vi "Process.vi"(9 "process sync":refnum<notifier>, 11 "DAQ_Engine in":refnum<class "DAQ_Engine.lvclass">) -> ()   [LabVIEW 2019, in "DAQ_Engine.lvclass"]
doc: "Developed by Kevin Thompson\nkevin@thompsonengineering.net\n\nCopyright 2018\nThompson Engineering, LLC"
uses:
  DAQ_Engine.lvclass
  Common/DataTypes/Measurement Config--cluster.ctl
  DataTypes/DAQLoopSMcase--enum.ctl
  DataTypes/Process - AppData--cluster.ctl
  DataTypes/Settings--cluster.ctl
  Common/DataTypes/Acquisition Mode--cluster.ctl
  DataTypes/Dependency--cluster.ctl
  Config/Config.lvclass
  DataTypes/Public Events--cluster.ctl
  Common/DataTypes/TD Async CmdMsg EventData--cluster.ctl
  DataTypes/DAQStateChg EvData--cluster.ctl
  DataTypes/DAQStateEvData--cluster.ctl
  Common/DataTypes/DAQState--enum.ctl
  DataTypes/DAQMeasSettingsChg EvData--cluster.ctl
  DataTypes/DAQMeasSettingsEvData--cluster.ctl
  DataTypes/DAQAcqModeChg EvData--cluster.ctl
  Common/DataTypes/RawDAQDataQRef--cluster.ctl
  Common/DataTypes/RawDAQData--cluster.ctl
  Common/DataTypes/RawChannelData--cluster.ctl
  Common/DataTypes/TD GetSet ActionSelect--enum.ctl
  DAQ_Engine.lvclass/DAQ_Engine.ctl
  DataTypes/PrivateAsynEv_DAQ_Engine--enum.ctl
  Accessors/Get Settings.vi
  Accessors/Get PublicEvents.vi
  Accessors/Get Dependency.vi
  Accessors/Get RawDaqDataQRef.vi
  Accessors/Get ObjData.vi
  Accessors/Set MeasSettings.vi
  Accessors/Set InverterDataAcqMode.vi
  Accessors/Get MeasSettings.vi
  Accessors/Get InverterDataAcqMode.vi
  <vilib>/TELLC/SMQ/Add States to Queue using MultiLine String with vData.vi
  Common/Startup/GBL System.vi
panel:
  out "WaitFunction Value":u32
  out "computed loop time":u32
  out "ErrReporting":i32
  out "DAQ Error":bool
  out "DaqQ Timeout":bool
  in  "MeasSet":T1={"Data Rate 9775"=3.0, "Data Rate 9215"=1200000.0, "Samples RMS 9215"=480000, "Samples RMS 9775"=3}
  out "QuitSense":bool
  in  "HSLoopEn":bool
  in  "Enable DAQ":bool
  in  "Exit":bool
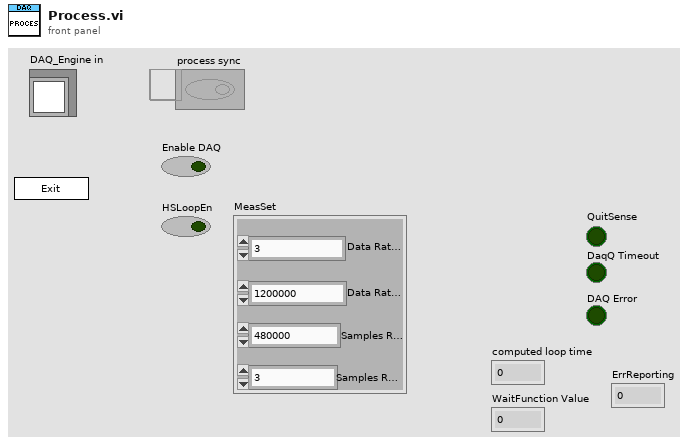
[diagram p1: front panel]
types:
  T1 = typedef "Measurement Config--cluster.ctl" = cluster{"Data Rate 9775":dbl, "Data Rate 9215":dbl, "Samples RMS 9215":u32, "Samples RMS 9775":u32}
  T2 = typedef "DAQ_Engine.lvclass/DAQLoopSMcase--enum.ctl" = enum16{"Init", "Run", "Stop"}
  T3 = typedef "TD GetSet ActionSelect--enum.ctl" = enum16{"Init", "Get", "Set"}
  T4 = typedef "DAQState--enum.ctl" = enum16{"Unknown", "Stopped", "Running", "Error"}
  T5 = typedef "DAQ_Engine.lvclass/Process - AppData--cluster.ctl" = cluster{"Core":cluster{"Current VI Reference":refnum<vi>, "Close Panel on Exit?":bool}, "Your Boolean data":bool, "Your string data":string, "SMQ":refnum<queue>, "Initialized?":bool, "Self Reference":refnum<class "DAQ_Engine.lvclass">, "Simulation?":bool, "process sync":refnum<notifier>, "vData":variant, "Settings":T6, "Dependency":T8, "Public Events":T9, "RawDaqDataQ":T10, "PrivateAsync Ev":refnum<user-event>, "MeasSet":T1, "AcqMode":T7, "DAQState Data":T11}
  T6 = typedef "DAQ_Engine.lvclass/Settings--cluster.ctl" = cluster{"Simulation":bool, "Initial ErrReporting setting":i32, "Initial Measurement settings":T1, "Acquisition mode":T7, "DemoMode":bool, "RIO Device":string}
  T7 = typedef "Acquisition Mode--cluster.ctl" = enum16{"3phase", "Single"}
  T8 = typedef "DAQ_Engine.lvclass/Dependency--cluster.ctl" = cluster{"Config":refnum<class "Config.lvclass">}
  T9 = typedef "DAQ_Engine.lvclass/Public Events--cluster.ctl" = cluster{"DAQ_Engine.AsyncCmd Event":refnum<user-event>, "DAQ_Engine.AsyncMsg Event":refnum<user-event>, "stop process":refnum<user-event>, "DAQ_Engine.DAQStateChg Ev":refnum<user-event>, "DAQ_Engine.MeasSettingsChg Ev":refnum<user-event>, "DAQ_Engine.AcqModeChg Ev":refnum<user-event>}
  T10 = typedef "RawDAQDataQRef--cluster.ctl" = refnum<queue>
  T11 = typedef "DAQ_Engine.lvclass/DAQStateEvData--cluster.ctl" = cluster{"DAQState":T4, "vData":variant}
  T12 = typedef "DAQ_Engine.lvclass/ObjData--cluster.ctl" = cluster{"Settings":T6, "Public Events":T9, "Dependency":T8, "ReadData-placeholder":T13, "VISA-placeholder":refnum<visa-resource-name>, "MeasSettings":T1, "InverterDataAcqMode":T7, "RawDaqDataQ":T10, "Private Events":T14, "DAQState Data":T11}
  T13 = typedef "DAQ_Engine.lvclass/Read Data--cluster.ctl" = cluster{"Data":dbl}
  T14 = typedef "DAQ_Engine.lvclass/Private Events--cluster.ctl" = cluster{"PrivateAsync Ev":refnum<user-event>}
  T15 = typedef "DAQ_Engine.lvclass/PrivateAsynEv_DAQ_Engine--enum.ctl" = enum16{"PrivDAQ.EnableDAQ", "PrivDAQ.ClearDAQError"}
  T16 = enum32{"invalid app kind", "Development System", "Run Time System", "Student Edition", "Embedded LabVIEW", "Evaluation", "Custom"}
  T17 = enum32{"Invalid", "Standard", "Closed", "Hidden", "Minimized", "Maximized"}
  T18 = typedef "DAQ_Engine.lvclass/AsynCmd_DAQ_Engine--enum.ctl" = enum16{"DAQ.EnableDAQ", "DAQ.ClearDAQError", "DAQ.SetMeasConfig", "DAQ.SetAcqMode", "DAQ.SetErrorReporting"}
  T19 = cluster{"Current VI Reference":refnum<vi>, "Close Panel on Exit?":bool}
  T20 = typedef "RawDAQData--cluster.ctl" = cluster{"Module1-2_9775":T21, "Module 3-4_9215":T21}
  T21 = typedef "RawChannelData--cluster.ctl" = cluster{"TS":timestamp, "ScanArray":dbl[]}
  T22 = typedef "nirio_resource_hc.ctl" = tag
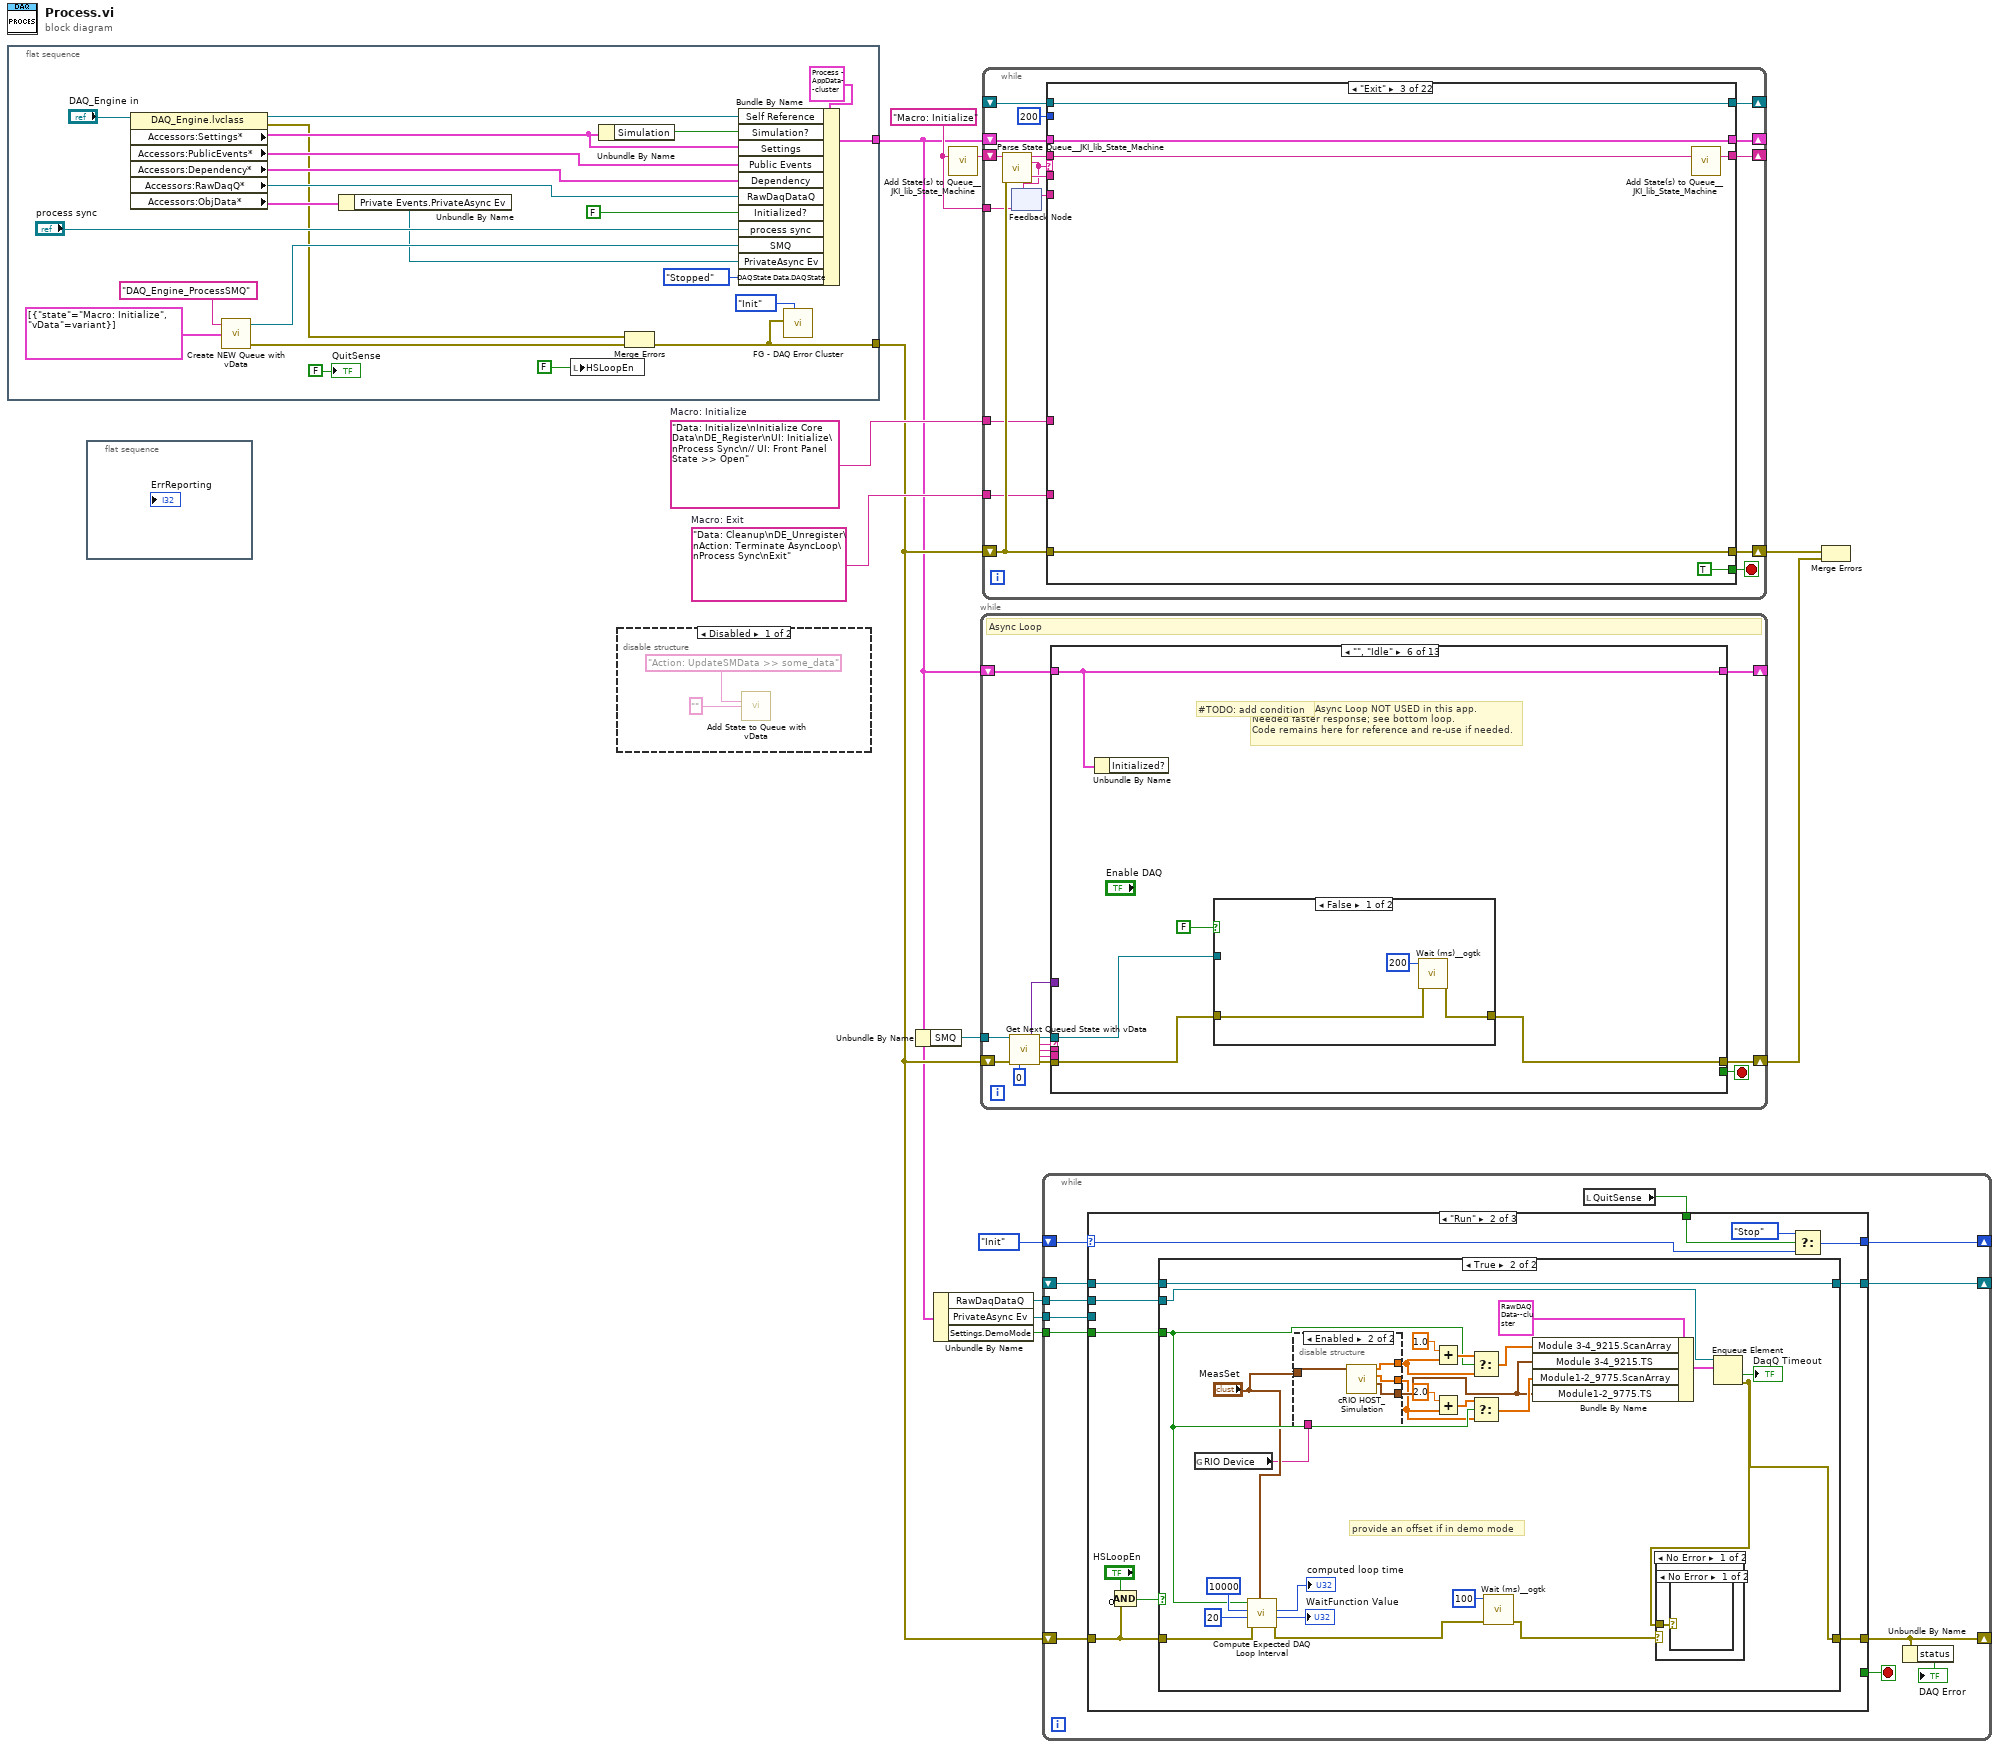
[diagram p0: block diagram]
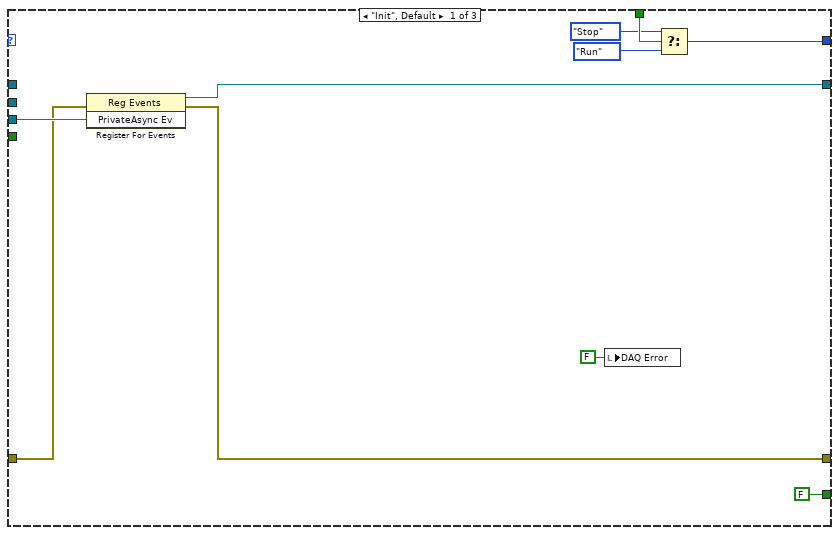
[diagram p2: hidden frame]
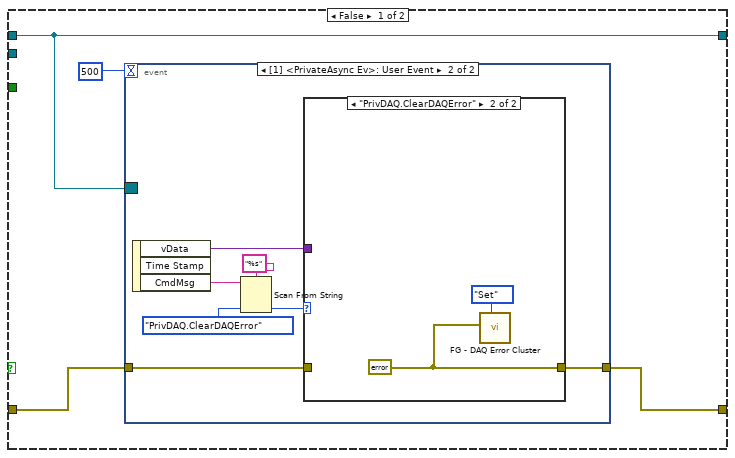
[diagram p3: hidden frame]
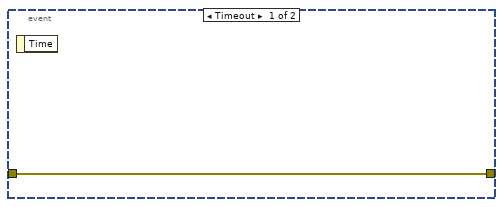
[diagram p4: hidden frame]
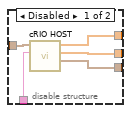
[diagram p6: hidden frame]
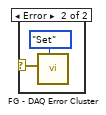
[diagram p7: hidden frame]
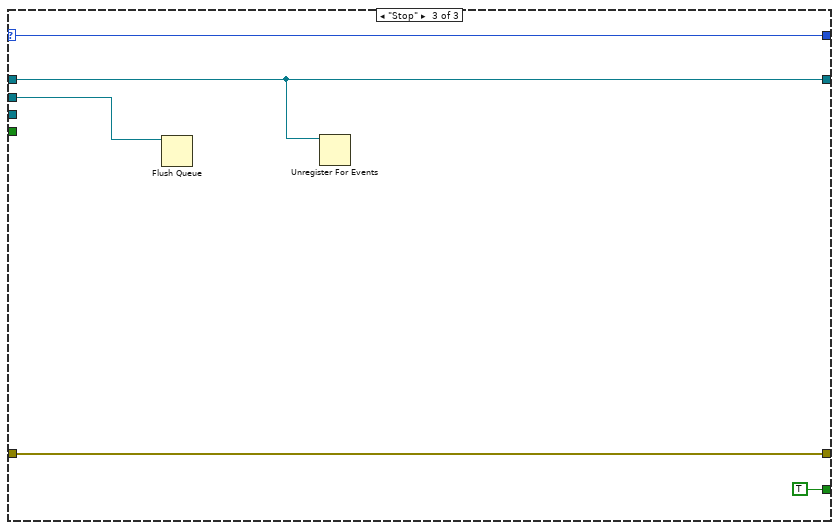
[diagram p9: hidden frame]
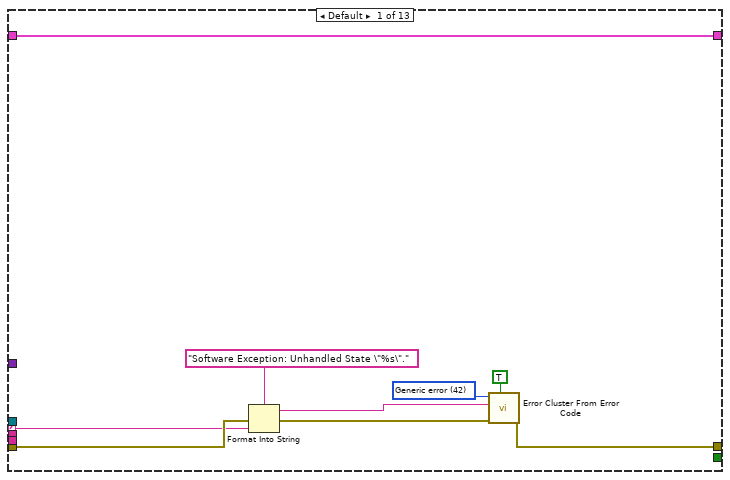
[diagram p11: hidden frame]
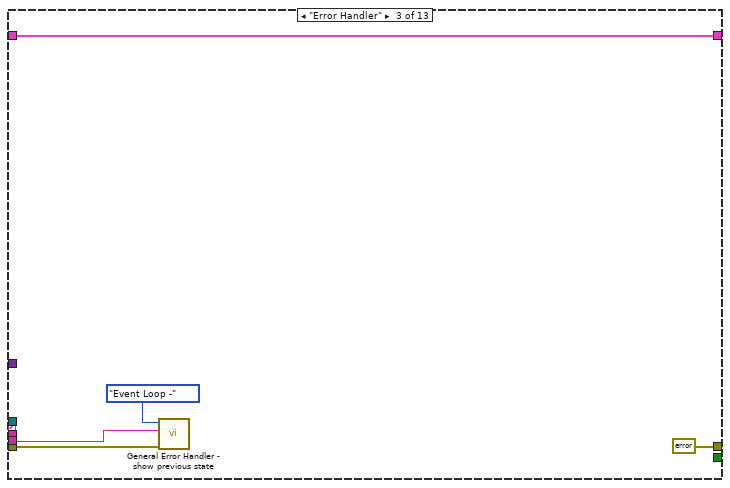
[diagram p13: hidden frame]
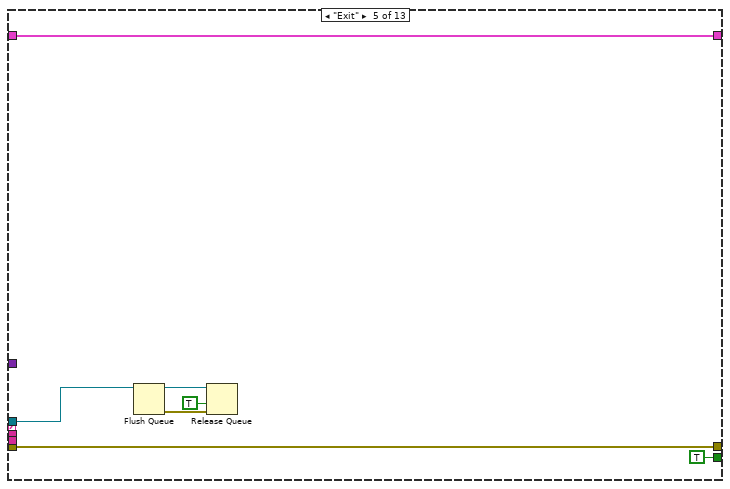
[diagram p15: hidden frame]
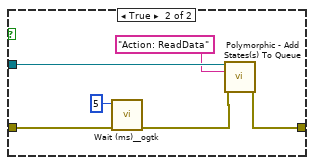
[diagram p16: hidden frame]
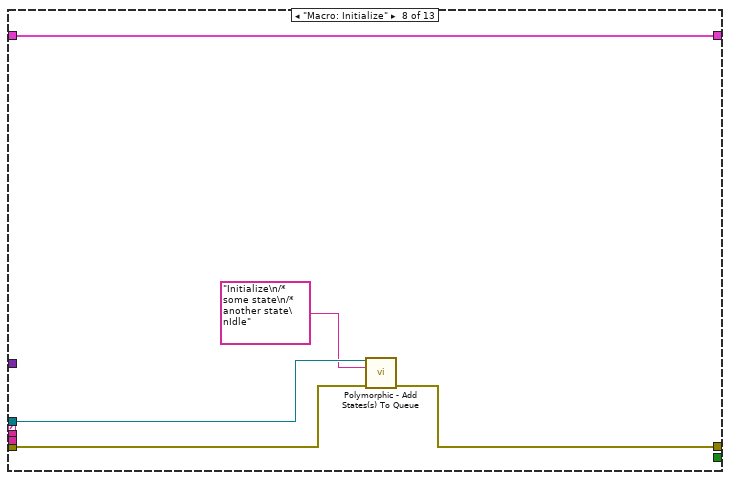
[diagram p18: hidden frame]
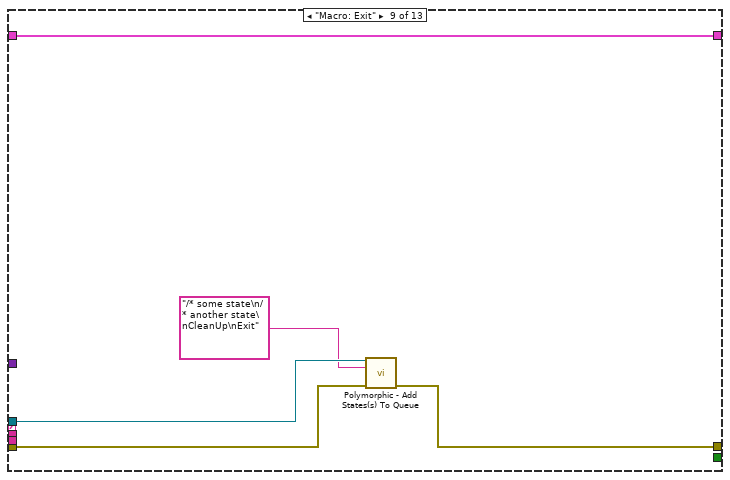
[diagram p19: hidden frame]
diagram:
  w11 = "Data: Cleanup\nDE_Unregister\nAction: Terminate AsyncLoop\nProcess Sync\nExit"  # Macro: Exit
  w12 = "Data: Initialize\nInitialize Core Data\nDE_Register\nUI: Initialize\nProcess Sync\n// UI: Front Panel State >> Open"  # Macro: Initialize
  w7 = "Macro: Initialize"
  n1 = flat-sequence {
    tunnel: [w36] -> w4
    tunnel: [w15] -> w5
    frame #0 {
      n2 = property class="DAQ_Engine.lvclass"(reference="DAQ_Engine in") -> (reference out=w17:refnum<class "DAQ_Engine.lvclass">, error out=w16:errorcluster, "Accessors:Settings*"=w27:T6, "Accessors:PublicEvents*"=w18:T9, "Accessors:Dependency*"=w29:T8, "Accessors:RawDaqQ*"=w23:T10, "Accessors:ObjData*"=w22:T12)  [unwired: 1 in]
      n3 = call <vilib>:"Create NEW Queue with vData.vi"("Initial States"=cluster{"state":string, "vData":variant}[] [{"state"="Macro: Initialize", "vData"=variant}], "Name (SMQ)"="DAQ_Engine_ProcessSMQ") -> ("error out"=w19:errorcluster, "queue out"=w35:refnum<queue>)  [unwired: 2 in]
      n4 = Unbundle By Name(w22) -> ("Private Events.PrivateAsync Ev"=w21:refnum<user-event>)
      n5 = local write "HSLoopEn"(FALSE ("HSLoopEn")) -> ()
      n6 = Unbundle By Name(w27) -> ("Simulation"=w28:bool)
      n7 = Merge Errors(w16, w19) -> (w15:errorcluster)
      n8 = Bundle By Name(cluster=T5 {"Core"={"Current VI Reference"=refnum, "Close Panel on Exit?"=FALSE}, "Your Boolean data"=FALSE, "Your string data"="", "SMQ"=refnum, "Initialized?"=FALSE, "Self Reference"=refnum, "Simulation?"=FALSE, "process sync"=refnum, "vData"=variant, "Settings"={"Simulation"=FALSE, "Initial ErrReporting setting"=0, "Initial Measurement settings"={"Data Rate 9775"=3.0, "Data Rate 9215"=1200000.0, "Samples RMS 9215"=480000, "Samples RMS 9775"=3}, "Acquisition mode"=enum."3phase", "DemoMode"=FALSE, "RIO Device"=""}, "Dependency"={"Config"=refnum}, "Public Events"={"DAQ_Engine.AsyncCmd Event"=refnum, "DAQ_Engine.AsyncMsg Event"=refnum, "stop process"=refnum, "DAQ_Engine.DAQStateChg Ev"=refnum, "DAQ_Engine.MeasSettingsChg Ev"=refnum, "DAQ_Engine.AcqModeChg Ev"=refnum}, "RawDaqDataQ"=refnum, "PrivateAsync Ev"=refnum, "MeasSet"={"Data Rate 9775"=3.0, "Data Rate 9215"=1200000.0, "Samples RMS 9215"=480000, "Samples RMS 9775"=3}, "AcqMode"=enum."3phase", "DAQState Data"={"DAQState"=enum."Unknown", "vData"=variant}} ("SM2 AppData"), "Self Reference"=w17, "Simulation?"=w28, "Settings"=w27, "Public Events"=w18, "Dependency"=w29, "RawDaqDataQ"=w23, "Initialized?"=FALSE, "process sync"="process sync", "SMQ"=w35, "PrivateAsync Ev"=w21, "DAQState Data.DAQState"=DAQState--enum."Stopped") -> (w36:T5)
      n9 = call "FG - DAQ Error Cluster.vi"("action (Get)"=TD_GetSet_ActionSelect--enum."Init", "error"=w15) -> ()  [unwired: 9 in, 1 out]
      "QuitSense" <- FALSE ("QuitSense")
    }
  }
  n10 = flat-sequence {
    frame #0 {
    }
  }
  n11 = disable-structure shown="Disabled" {
    frame Disabled {
      n12 = call <vilib>:"Add State to Queue with vData.vi"("state in"="Action: UpdateSMData >> some_data", "vData (\"\")"="") -> ()  [unwired: 10 in, 4 out]
    }
    frame Enabled {
    }
  }
  n13 = Unbundle By Name(w4) -> ("SMQ"=w10:refnum<queue>)
  n14 = Unbundle By Name(w4) -> ("RawDaqDataQ"=w6:T10, "PrivateAsync Ev"=w2:refnum<user-event>, "Settings.DemoMode"=w1:bool)
  n15 = call <vilib>:"Add State(s) to Queue__JKI_lib_State_Machine.vi"("State(s) in (\"\")"=w7) -> ("States Out"=w13:string)  [unwired: 14 in]
  n16 = while {
    shift-right: [w48] -> w8
    shift-left: w5 -> [w50]
    tunnel: w10 -> [w46]
    shift-right: [w44] -> _
    shift-left: w4 -> [w45]
    stop <- w39 stop-if-true
    # "Async Loop"
    n17 = call <vilib>:"Get Next Queued State with vData.vi"("queue in"=w46, "error in (no error)"=w50, "timeout (100)"=0) -> ("vData out"=w43:variant, "queue out"=w47:refnum<queue>, "Next State"=w51:string, "queued msg"=w41:string, "Prev State"=w40:string, "error out"=w49:errorcluster)  [unwired: 6 in, 1 out]
    n18 = case shown="\"\", \"Idle\"" w51 {
      tunnel: w47 -> [_ _ _ _ w70 w81 _ w96 w101 _ _ _ w120]
      tunnel: w41 -> [_ _ _ _ _ _ _ _ _ _ _ w109 w122]
      selector: w51 -> [w52 _ _ _ _ _ _ _ _ _ _ _ _]
      tunnel: w49 -> [w54 w62 w64 w69 w76 w78 w92 w95 w100 w104 w105 w108 w117]
      tunnel: [w53 w62 errorcluster {"status"=FALSE, "code"=0, "source"=""} ("error constant") w69 w76 w79 w92 w94 w99 w104 w105 w111 w116] -> w48
      tunnel: w45 -> [w60 w61 w67 w68 w75 w80 w91 w97 w102 w103 w106 w114 w119]
      tunnel: [w60 w61 w67 w68 w75 w80 w91 w97 w102 w103 w106 w114 w118] -> w44
      tunnel: w43 -> [_ _ _ _ _ _ _ _ _ _ _ _ w121]
      tunnel: w40 -> [_ _ w63 _ _ _ _ _ _ _ _ _ _]
      tunnel: [_ _ _ _ TRUE _ _ _ _ _ _ _ _] -> w39
      frame Default {
        w56 = 42 items=["No error", "Argument error", "Memory is full", "Out of zone", "End of file", "File already open", "Generic file I/O error", "File not found", "File permission error", "Disk is full", "Duplicate path", "Too many files open", "System feature not enabled", "Resource file not found", "Cannot add resource", "Resource not found", "Image not found", "Image memory error", "Pen does not exist", "Config type invalid", "Config token not found", "Config parse error", "Config memory error", "Bad external code format", "Bad external code offset", "External code not present", "Null window", "Destroy window error", "Null menu", "Print aborted", "Bad print record", "Print driver error", "Windows error during printing", "Memory error during printing", "Print dialog error", "Generic print error", "Invalid device refnum", "Device not found", "Device parameter error", "Device unit error", "Cannot open device", "Device call aborted", "Generic error", "Cancelled by user", "Object ID too low", "Object ID too high", "Object not in heap", "Unknown heap", "Unknown object (invalid DefProc)", "Unknown object (DefProc not in table)", "Message out of range", "Invalid (null) method", "Unknown message", "Manager call not supported", "Bad address", "Network operation in progress", "Network operation timed out", "Connection is busy", "Network attribute not supported", "Network error", "Address in use", "System out of memory", "Connection aborted", "Connection refused", "Not connected", "Already connected", "Connection closed", "Initialization error (interapplication manager)", "Bad occurrence", "Wait on unbound occurrence handler", "Occurrence queue overflow", "Datalog type conflict", "Unused", "Unrecognized type (interapplication manager)", "Memory corrupt", "Failed to make temporary DLL", "Old CIN version", "Drag socket not found", "Failed to load drop-object", "Failed to register OLE object", "Failed to release OLE object", "Format specifier type mismatch", "Unknown format specifier", "Too few format specifiers", "Too many format specifiers", "Scan failed", "Newer CIN version", "Error converting to variant", "Runtime menu error", "Password tampered", "Variant attribute not found", "Incompatible variant data type", "Event data is not available", "Event Store is not present", "Occurrence is not found", "Event Queue is not created", "Event info is not available", "Refnum passed is NULL", "Error retrieving Class GUID", "Error retrieving CoClass GUID", "Error retrieving TypeLib GUID.", "Bad built application magic bytes.", "Specific driver is different from the specific driver associated with the Logical Name.", "There is no session opened to the class driver.", "Max Error", "MAX - Error with config objects", "MAX - Error loading configuration", "MAX - Group not supported"]
        n19 = Format Into String(format string="Software Exception: Unhandled State \"%s\"." ("message"), error in=w54, w52) -> (resulting string=w57:string, error out=w58:errorcluster)  [unwired: 1 in]
        n20 = call <vilib>:"Error Cluster From Error Code.vi"("show call chain? (False)"=TRUE, "error in (no error)"=w58, "error message (\"\")"=w57, "error code (0)"=w56) -> ("error out"=w53:errorcluster)  [unwired: 5 in]
      }
      frame "Initialize" {
      }
      frame "Error Handler" {
        n21 = call "General Error Handler - show previous state.vi"("error in (no error)"=w64, "Previous State"=w63, "Loop Select"=enum16{"Event Loop -", "Async Loop -"}."Event Loop -") -> ()  [unwired: 7 in, 2 out]
      }
      frame "CleanUp" {
      }
      frame "Exit" {
        n22 = Flush Queue(queue=w70) -> (queue out=w73:refnum<queue>, error out=w72:errorcluster)  [unwired: 1 in, 1 out]
        n23 = Release Queue(queue=w73, force destroy? (F)=TRUE, error in (no error)=w72) -> ()  [unwired: 3 out]
      }
      frame "", "Idle" {
        # "#NOTE: This Async Loop NOT USED in this app.\nNeeded faster response; see bottom loop.\nCode remains here for reference and re-use if needed."
        # "#TODO: add condition"
        n24 = Unbundle By Name(w80) -> ()  [unwired: 1 out]
        n25 = case shown="False" FALSE {
          tunnel: w81 -> [_ w90]
          tunnel: w78 -> [w82 w88]
          tunnel: [w83 w85] -> w79
          frame False {
            n26 = call <userlib>:"Wait (ms)__ogtk.vi"("error in (no error)"=w82, "milliseconds to wait"=u32 200) -> ("error out"=w83:errorcluster)  [unwired: 8 in, 1 out]
          }
          frame True {
            n27 = call <userlib>:"Wait (ms)__ogtk.vi"("error in (no error)"=w88, "milliseconds to wait"=u32 5) -> ("error out"=w86:errorcluster)  [unwired: 8 in, 1 out]
            n28 = call-poly <vilib>:"Polymorphic - Add States(s) To Queue.vi"("queue in"=w90, "state in"="Action: ReadData", "error in"=w86) -> ("error out"=w85:errorcluster)  [unwired: 9 in, 3 out]
          }
        }
      }
      frame "------ Macro ------" {
      }
      frame "Macro: Initialize" {
        n29 = call-poly <vilib>:"Polymorphic - Add States(s) To Queue.vi"("queue in"=w96, "states in"="Initialize\n/* some state\n/* another state\nIdle", "error in"=w95) -> ("error out"=w94:errorcluster)  [unwired: 10 in, 2 out]
      }
      frame "Macro: Exit" {
        n30 = call-poly <vilib>:"Polymorphic - Add States(s) To Queue.vi"("queue in"=w101, "states in"="/* some state\n/* another state\nCleanUp\nExit", "error in"=w100) -> ("error out"=w99:errorcluster)  [unwired: 10 in, 2 out]
      }
      frame "------ Action ------" {
      }
      frame "Action: ReadData" {
        # "do nothing"
      }
      frame "Action: Wait" {
        n31 = Scan From String(format string="%d", input string=w109, error in=w108, default 1=u32 0) -> (error out=w107:errorcluster, output 1=w113:u32)  [unwired: 1 in, 2 out]
        n32 = call <userlib>:"Wait (ms)__ogtk.vi"("error in (no error)"=w107, "milliseconds to wait"=w113) -> ("error out"=w111:errorcluster)  [unwired: 8 in, 1 out]
      }
      frame "Action: UpdateSMData" {
        n33 = Match Pattern(string=w122, regular expression=":") -> (before substring=w124:string, after substring=w115:string)  [unwired: 1 in, 2 out]
        n34 = case shown="\"some_data\"" w124 {
          tunnel: w121 -> [_ w131]
          tunnel: w120 -> [_ _]
          tunnel: w119 -> [w125 w130]
          tunnel: [w125 w129] -> w118
          tunnel: w117 -> [w126 w128]
          tunnel: [w126 w127] -> w116
          tunnel: w115 -> [_ _]
          frame Default {
            # "#NOTE:\noptionally add error here."
          }
          frame "some_data" {
            n35 = disable-structure shown="Disabled" {
              disable-tunnel: w131 -> [w138 _]
              disable-tunnel: w128 -> [w136 w139]
              disable-tunnel: [w135 w139] -> w127
              frame Disabled {
                n36 = Variant To Data(error in=w136, type="", Variant=w138) -> (error out=w135:errorcluster)  [unwired: 1 out]
              }
              frame Enabled {
              }
            }
            n37 = disable-structure shown="Disabled" {
              disable-tunnel: w130 -> [w133 w134]
              disable-tunnel: [w132 w134] -> w129
              frame Disabled {
                n38 = Bundle By Name(cluster=w133) -> (w132:T5)  [unwired: 1 in]
              }
              frame Enabled {
              }
            }
          }
        }
      }
    }
  }
  n39 = while {
    shift-right: [w150] -> _
    shift-left: w4 -> [w149]
    shift-right: [w153] -> w9
    shift-left: w5 -> [w148]
    shift-right: [w152] -> _
    shift-left: w13 -> [w154]
    shift-right: [w147] -> _
    shift-left: _ -> [w146]
    tunnel: w12 -> [w144]
    tunnel: w11 -> [w143]
    tunnel: w7 -> [w142]
    stop <- w151 stop-if-true
    n40 = call <vilib>:"Parse State Queue__JKI_lib_State_Machine.vi"("State Queue"=w154, "Error In (no error)"=w148) -> ("Remaining States"=w156:string, "Current State"=w141:string, "Arguments"=w155:string)  [unwired: 11 in]
    n41 = feedback #1(w142) -> (w140:string)
    n42 = feedback-in #1(w141) -> ()
    n43 = case shown="\"Exit\"" w141 {
      selector: w141 -> [w158 _ _ _ _ _ _ _ _ _ _ _ _ _ _ _ _ _ _ _ _ _]
      tunnel: w156 -> [w162 w177 w183 w191 w305 w318 w326 w331 w335 w340 w349 w356 w361 w374 w385 w397 w424 w430 w442 w447 w458 w467]
      tunnel: w155 -> [_ _ _ _ _ _ _ _ _ _ _ _ _ _ w380 w391 _ _ _ _ w448 _]
      tunnel: w149 -> [w160 w174 w178 w189 w302 w309 w323 w328 w334 w337 w341 w351 w358 w363 w383 w393 w421 w427 w439 w444 w456 w464]
      tunnel: [w164 errorcluster {"status"=FALSE, "code"=0, "source"=""} ("error out") w181 w188 w303 w315 w319 w329 w332 w338 w347 w352 w359 w368 w381 w394 w422 w428 w440 w445 w449 w459] -> w153
      tunnel: w148 -> [w163 w170 w181 w187 w303 w315 w320 _ w332 w338 w347 w353 w359 w371 w382 w395 w422 w428 w440 w445 w450 w460]
      tunnel: [w161 w176 w182 w190 w304 w317 w325 w331 w335 w339 w348 w355 w360 w373 w384 w396 w423 w429 w441 w446 w457 w466] -> w152
      tunnel: [_ _ TRUE _ _ _ _ _ _ _ _ _ _ _ _ _ _ _ _ _ _ _] -> w151
      tunnel: [w160 w174 w178 w186 w302 w316 w323 w328 w334 w337 w343 w351 w358 w364 w383 w393 w421 w427 w439 w444 w456 w464] -> w150
      tunnel: [w157 w172 w179 w184 w301 w306 w324 w330 w333 w336 w342 w350 w357 w372 w379 w390 w420 w426 w433 w443 w455 w465] -> w147
      tunnel: w146 -> [w157 w172 w179 w184 w301 w306 w324 _ w333 w336 w342 w350 w357 w372 w379 w390 w420 w426 w433 w443 w455 w465]
      tunnel: 200 ("Timeout") -> [_ _ _ w185 _ _ _ _ _ _ _ _ _ _ _ _ _ _ _ _ _ _]
      tunnel: w144 -> [_ _ _ _ _ _ _ _ _ _ _ _ _ _ _ _ _ w425 _ _ _ _]
      tunnel: w143 -> [_ _ _ _ _ _ _ _ _ _ _ _ _ _ _ _ _ _ w432 _ _ _]
      tunnel: w140 -> [_ w169 _ _ _ _ _ _ _ _ _ _ _ _ _ _ _ _ _ _ _ _]
      frame Default {
        w167 = 42 items=["No error", "Argument error", "Memory is full", "Out of zone", "End of file", "File already open", "Generic file I/O error", "File not found", "File permission error", "Disk is full", "Duplicate path", "Too many files open", "System feature not enabled", "Resource file not found", "Cannot add resource", "Resource not found", "Image not found", "Image memory error", "Pen does not exist", "Config type invalid", "Config token not found", "Config parse error", "Config memory error", "Bad external code format", "Bad external code offset", "External code not present", "Null window", "Destroy window error", "Null menu", "Print aborted", "Bad print record", "Print driver error", "Windows error during printing", "Memory error during printing", "Print dialog error", "Generic print error", "Invalid device refnum", "Device not found", "Device parameter error", "Device unit error", "Cannot open device", "Device call aborted", "Generic error", "Cancelled by user", "Object ID too low", "Object ID too high", "Object not in heap", "Unknown heap", "Unknown object (invalid DefProc)", "Unknown object (DefProc not in table)", "Message out of range", "Invalid (null) method", "Unknown message", "Manager call not supported", "Bad address", "Network operation in progress", "Network operation timed out", "Connection is busy", "Network attribute not supported", "Network error", "Address in use", "System out of memory", "Connection aborted", "Connection refused", "Not connected", "Already connected", "Connection closed", "Initialization error (interapplication manager)", "Bad occurrence", "Wait on unbound occurrence handler", "Occurrence queue overflow", "Datalog type conflict", "Unused", "Unrecognized type (interapplication manager)", "Memory corrupt", "Failed to make temporary DLL", "Old CIN version", "Drag socket not found", "Failed to load drop-object", "Failed to register OLE object", "Failed to release OLE object", "Format specifier type mismatch", "Unknown format specifier", "Too few format specifiers", "Too many format specifiers", "Scan failed", "Newer CIN version", "Error converting to variant", "Runtime menu error", "Password tampered", "Variant attribute not found", "Incompatible variant data type", "Event data is not available", "Event Store is not present", "Occurrence is not found", "Event Queue is not created", "Event info is not available", "Refnum passed is NULL", "Error retrieving Class GUID", "Error retrieving CoClass GUID", "Error retrieving TypeLib GUID.", "Bad built application magic bytes.", "Specific driver is different from the specific driver associated with the Logical Name.", "There is no session opened to the class driver.", "Max Error", "MAX - Error with config objects", "MAX - Error loading configuration", "MAX - Group not supported"]
        # "Current State"
        n44 = Format Into String(format string="Software Exception: Unhandled State \"%s\"." ("message"), error in=w163, w158) -> (resulting string=w166:string, error out=w165:errorcluster)  [unwired: 1 in]
        n45 = call <vilib>:"Error Cluster From Error Code.vi"("show call chain? (False)"=TRUE, "error in (no error)"=w165, "error message (\"\")"=w166, "error code (0)"=w167) -> ("error out"=w164:errorcluster)  [unwired: 5 in]
        n46 = call <vilib>:"Add State(s) to Queue__JKI_lib_State_Machine.vi"("State(s) in (\"\")"=w162) -> ("States Out"=w161:string)  [unwired: 14 in]
      }
      frame "Error Handler" {
        n47 = call "General Error Handler - show previous state.vi"("error in (no error)"=w170, "Previous State"=w169, "Loop Select"=enum16{"Event Loop -", "Async Loop -"}."Event Loop -") -> ()  [unwired: 7 in, 2 out]
        n48 = call <vilib>:"Add State(s) to Queue__JKI_lib_State_Machine.vi"("State(s) in Front (\"\")"="/* Post Error States", "State(s) in (\"\")"=w177) -> ("States Out"=w176:string)  [unwired: 13 in]
      }
      frame "Exit" {
        n49 = call <vilib>:"Add State(s) to Queue__JKI_lib_State_Machine.vi"("State(s) in (\"\")"=w183) -> ("States Out"=w182:string)  [unwired: 14 in]
      }
      frame "", "Event Structure", "Idle" {
        n50 = event shown="[5] <Public Events.DAQ_Engine.AsyncCmd Event>: User Event" {
          selector: w184 -> [_ _ _ _ _ _]
          dyn-events: _ -> [_ _ _ _ _ _]
          timeout: w185 -> [_ _ _ _ _ _]
          tunnel: w191 -> [w195 w200 w206 w209 w216 w232]
          tunnel: [w194 w199 w205 w208 w215 w231] -> w190
          tunnel: w189 -> [w192 w197 w203 w211 w219 w221]
          tunnel: [w193 w198 w204 w212 w220 w229] -> w188
          tunnel: w187 -> [w193 w198 w204 w212 w220 w228]
          tunnel: [w192 w197 w203 w211 w218 w223] -> w186
          event Timeout {
            n51 = event-data() -> ()  [unwired: 1 in, 1 out]
            n52 = call <vilib>:"Add State(s) to Queue__JKI_lib_State_Machine.vi"("State(s) in (\"\")"=w195) -> ("States Out"=w194:string)  [unwired: 14 in]
          }
          event "Exit": Value Change {
            n53 = event-data() -> ()  [unwired: 1 in, 1 out]
            n54 = call <vilib>:"Add State(s) to Queue__JKI_lib_State_Machine.vi"("State(s) in Front (\"\")"="Macro: Exit", "State(s) in (\"\")"=w200) -> ("States Out"=w199:string)  [unwired: 13 in]
          }
          event Panel Close? {
            n55 = event-data() -> ()  [unwired: 1 in, 1 out]
            n56 = event-data("Discard?"=TRUE) -> ()  [unwired: 1 in, 1 out]
            n57 = call <vilib>:"Add State(s) to Queue__JKI_lib_State_Machine.vi"("State(s) in Front (\"\")"="Macro: Exit", "State(s) in (\"\")"=w206) -> ("States Out"=w205:string)  [unwired: 13 in]
          }
          event Menu Selection (User) {
            n58 = event-data() -> ("ItemTag"=w210:string)  [unwired: 1 in, 2 out]
            n59 = case shown="\"False\", Default" w210 {
              tunnel: [""] -> w207
              frame "False", Default {
              }
            }
            n60 = call <vilib>:"Add State(s) to Queue__JKI_lib_State_Machine.vi"("State(s) in Front (\"\")"=w207, "State(s) in (\"\")"=w209) -> ("States Out"=w208:string)  [unwired: 13 in]
          }
          event User Event {
            n61 = event-data() -> ("notifier out"=w217:refnum<notifier>)  [unwired: 1 in]
            n62 = Bundle By Name(cluster=w219, "process sync"=w217) -> (w218:T5)
            n63 = call <vilib>:"Add State(s) to Queue__JKI_lib_State_Machine.vi"("State(s) in Front (\"\")"="Macro: Exit", "State(s) in (\"\")"=w216) -> ("States Out"=w215:string)  [unwired: 13 in]
          }
          event User Event {
            n64 = event-data() -> ("CmdMsg"=w226:string, "vData"=w230:variant)  [unwired: 1 in, 1 out]
            n65 = Unbundle By Name(w221) -> ("Self Reference"=w222:refnum<class "DAQ_Engine.lvclass">)
            n66 = call "get async cmd.vi"("error in (no error)"=w228, "Cmd String in"=w226) -> ("error out"=w227:errorcluster, "AsyncCmd"=w225:T18)  [unwired: 8 in]
            n67 = case shown="\"DAQ.EnableDAQ\"" w225 {
              tunnel: w230 -> [_ w253 w263 w280 w293 w300]
              tunnel: w227 -> [w238 w252 w262 w279 w292 w299]
              tunnel: [w237 w240 w254 w269 w282 w297] -> w229
              tunnel: [_ "" "" "" "" ""] -> w224
              tunnel: w221 -> [w233 w250 w260 w277 w290 w294]
              tunnel: [w233 w249 w259 w276 w289 w294] -> w223
              tunnel: w222 -> [_ w248 w257 w273 w288 _]
              tunnel: w221 -> [_ _ _ _ _ _]
              frame Default {
                n68 = call <vilib>:"Build Error Cluster_ModKT .vi"("Prepend String (\"\")"="Invalid Async Cmd" ("Prepend String (\"\")"), "code"=42, "error? (F)"=TRUE, "error in (no error)"=w238) -> ("error out"=w237:errorcluster)  [unwired: 3 in, 1 out]
              }
              frame "DAQ.EnableDAQ" {
                n69 = Variant To Data(error in=w252, type=FALSE, Variant=w253) -> (data=w245:bool, error out=w241:errorcluster)
                n70 = Select(t=DAQState--enum."Running" ("DAQState Data.DAQState"), s=w245, f=DAQState--enum."Stopped") -> (s? t:f=w239:T4)
                n71 = local write "HSLoopEn"(w245) -> ()
                n72 = call "Fire DAQStateChanged Event_DAQ.vi"("error in (no error)"=w241, "vData"=variant, "DAQState"=w239, "DAQ_Engine in"=w248) -> ("error out"=w240:errorcluster)  [unwired: 6 in, 1 out]
                n73 = Bundle By Name(cluster=w250, "DAQState Data.DAQState"=w239, "DAQState Data.vData"=variant) -> (w249:T5)
              }
              frame "DAQ.ClearDAQError" {
                n74 = disable-structure shown="Disabled" {
                  disable-tunnel: w263 -> [w266 _]
                  disable-tunnel: w262 -> [w265 w267]
                  disable-tunnel: [w264 w267] -> w255
                  frame Disabled {
                    n75 = Variant To Data(error in=w265, Variant=w266) -> (error out=w264:errorcluster)  [unwired: 1 in, 1 out]
                  }
                  frame Enabled {
                  }
                }
                n76 = call "Fire Private Event.vi"("error in (no error)"=w255, "PrivAsyncCmd"=PrivateAsynEv_DAQ_Engine--enum."PrivDAQ.ClearDAQError", "DAQ_Engine in"=w257) -> ("error out"=w254:errorcluster)  [unwired: 7 in, 1 out]
                n77 = Bundle By Name(cluster=w260, "vData"=variant) -> (w259:T5)
              }
              frame "DAQ.SetMeasConfig" {
                n78 = Variant To Data(error in=w279, type=T1 {"Data Rate 9775"=3.0, "Data Rate 9215"=1200000.0, "Samples RMS 9215"=480000, "Samples RMS 9775"=3} ("MeasSet"), Variant=w280) -> (data=w271:T1, error out=w275:errorcluster)
                n79 = property class="DAQ_Engine.lvclass"(reference=w273, "Accessors:MeasSettings*"=w271) -> (reference out=w272:refnum<class "DAQ_Engine.lvclass">, error out=w270:errorcluster)  [unwired: 1 in]
                n80 = local write "MeasSet"(w271) -> ()
                n81 = call "Fire DAQMeasSettingsChanged Event_DAQ.vi"("error in (no error)"=w270, "Measurement config"=w271, "DAQ_Engine in"=w272) -> ("error out"=w268:errorcluster)  [unwired: 7 in, 1 out]
                n82 = Bundle By Name(cluster=w277, "MeasSet"=w271) -> (w276:T5)
                n83 = Merge Errors(w268, w275) -> (w269:errorcluster)
              }
              frame "DAQ.SetAcqMode" {
                n84 = Variant To Data(error in=w292, type=Acquisition_Mode--cluster."3phase" ("InverterDataAcqMode"), Variant=w293) -> (data=w285:T7, error out=w283:errorcluster)
                n85 = property class="DAQ_Engine.lvclass"(reference=w288, "Accessors:AcqMode*"=w285) -> (reference out=w286:refnum<class "DAQ_Engine.lvclass">, error out=w284:errorcluster)  [unwired: 1 in]
                n86 = Bundle By Name(cluster=w290, "AcqMode"=w285) -> (w289:T5)
                n87 = call "Fire DAQAcqModeChanged Event_DAQ.vi"("error in (no error)"=w284, "DAQState"=w285, "DAQ_Engine in"=w286) -> ("error out"=w281:errorcluster)  [unwired: 7 in, 1 out]
                n88 = Merge Errors(w281, w283) -> (w282:errorcluster)
              }
              frame "DAQ.SetErrorReporting" {
                n89 = Variant To Data(error in=w299, type=0 ("ErrReporting"), Variant=w300) -> (data=w295:i32, error out=w297:errorcluster)
                n90 = local write "ErrReporting"(w295) -> ()
                n91 = call "ErrHdlng.VI"("ErrReporting"=w295) -> ()  [unwired: 1 out]
              }
            }
            n92 = call <vilib>:"Add State(s) to Queue__JKI_lib_State_Machine.vi"("State(s) in Front (\"\")"=w224, "State(s) in (\"\")"=w232) -> ("States Out"=w231:string)  [unwired: 13 in]
          }
        }
      }
      frame "---------- Core ----------" {
        n93 = call <vilib>:"Add State(s) to Queue__JKI_lib_State_Machine.vi"("State(s) in (\"\")"=w305) -> ("States Out"=w304:string)  [unwired: 14 in]
      }
      frame "Initialize Core Data" {
        # "originally closed?"
        # "exe?"
        n94 = property class="VI"() -> ("Front Panel.Open"=w314:bool)  [unwired: 2 in, 2 out]
        n95 = property class="App"() -> ("App.Kind"=w313:T16)  [unwired: 2 in, 2 out]
        n96 = control-ref of="Current VI Reference"() -> (w307:refnum<vi>)
        n97 = Not(x=w314) -> (.not. x?=w311:bool)
        n98 = Equal?(x=w313, y=T16."Run Time System" ("Application:Kind")) -> (x = y?=w310:bool)
        n99 = Or(x=w311, y=w310) -> (x .or. y?=w308:bool)
        n100 = Bundle By Name(cluster=w309, "Core.Current VI Reference"=w307, "Core.Close Panel on Exit?"=w308) -> (w316:T5)
        n101 = call <vilib>:"Add State(s) to Queue__JKI_lib_State_Machine.vi"("State(s) in (\"\")"=w318) -> ("States Out"=w317:string)  [unwired: 14 in]
      }
      frame "Process Sync" {
        n102 = Unbundle By Name(w323) -> ("process sync"=w322:refnum<notifier>)
        n103 = Send Notification(notification=TRUE, notifier=w322, error in (no error)=w320) -> (error out=w319:errorcluster)  [unwired: 1 out]
        n104 = call <vilib>:"Add State(s) to Queue__JKI_lib_State_Machine.vi"("State(s) in (\"\")"=w326) -> ("States Out"=w325:string)  [unwired: 14 in]
      }
      frame "DE_Register" {
        n105 = Unbundle By Name(w328) -> ("Public Events"=w327:T9)
        n106 = register-events(w327) -> (reference out=w330:refnum<event-registration>, error out=w329:errorcluster)  [unwired: 2 in]
      }
      frame "DE_Unregister" {
        n107 = Unregister For Events(event registration refnum=w333, error in=w332) -> ()  [unwired: 1 out]
      }
      frame "---------- Data ----------" {
        n108 = call <vilib>:"Add State(s) to Queue__JKI_lib_State_Machine.vi"("State(s) in (\"\")"=w340) -> ("States Out"=w339:string)  [unwired: 14 in]
      }
      frame "Data: Initialize" {
        w344 = T19 {"Current VI Reference"=refnum, "Close Panel on Exit?"=FALSE}  # Core
        w346 = TRUE  # Your Boolean data
        w345 = ""  # Your string data
        n109 = Unbundle By Name(w341) -> ()  [unwired: 1 out]
        n110 = Bundle By Name(cluster=w341, "Core"=w344, "Your Boolean data"=w346, "Your string data"=w345) -> (w343:T5)
        n111 = call <vilib>:"Add State(s) to Queue__JKI_lib_State_Machine.vi"("State(s) in (\"\")"=w349) -> ("States Out"=w348:string)  [unwired: 14 in]
      }
      frame "Data: Cleanup" {
        n112 = Unbundle By Name(w351) -> ("Core.Current VI Reference"=w354:refnum<vi>)
        n113 = Close Reference(reference=w354, error in (no error)=w353) -> (error out=w352:errorcluster)
        n114 = call <vilib>:"Add State(s) to Queue__JKI_lib_State_Machine.vi"("State(s) in (\"\")"=w356) -> ("States Out"=w355:string)  [unwired: 14 in]
      }
      frame "---------- UI ----------" {
        n115 = call <vilib>:"Add State(s) to Queue__JKI_lib_State_Machine.vi"("State(s) in (\"\")"=w361) -> ("States Out"=w360:string)  [unwired: 14 in]
      }
      frame "UI: Initialize" {
        n116 = Unbundle By Name(w363) -> ("Settings.Initial ErrReporting setting"=w362:i32, "Self Reference"=w367:refnum<class "DAQ_Engine.lvclass">, "Core.Current VI Reference"=w370:refnum<vi>)
        n117 = disable-structure shown="Enabled" {
          disable-tunnel: w371 -> [w377 w378]
          disable-tunnel: w370 -> [w376 _]
          disable-tunnel: [w375 w378] -> w369
          frame Disabled {
            n118 = call <userlib>:"Fit VI window to Largest Dec__ogtk.vi"("error in (no error)"=w377, "VI Ref (calling VI)"=w376) -> ("error out"=w375:errorcluster)  [unwired: 4 in, 1 out]
          }
          frame Enabled {
          }
        }
        n119 = property class="DAQ_Engine.lvclass"(reference=w367, error in=w369) -> (error out=w368:errorcluster, "Accessors:MeasSettings*"=w366:T1, "Accessors:AcqMode*"=w365:T7)  [unwired: 1 out]
        n120 = local write "ErrReporting"(w362) -> ()
        n121 = call "ErrHdlng.VI"("ErrReporting"=w362) -> ()  [unwired: 1 out]
        n122 = local write "MeasSet"(w366) -> ()
        n123 = Bundle By Name(cluster=w363, "MeasSet"=w366, "AcqMode"=w365) -> (w364:T5)
        n124 = call <vilib>:"Add State(s) to Queue__JKI_lib_State_Machine.vi"("State(s) in (\"\")"=w374) -> ("States Out"=w373:string)  [unwired: 14 in]
      }
      frame "UI: Cursor Set" {
        # "Argument"
        n125 = case shown="\"Idle\", Default" w380 {
          tunnel: w382 -> [w387 w389]
          tunnel: [w386 w388] -> w381
          frame "Idle", Default {
            n126 = call <vilib>:"Unset Busy.vi"("error in (no error)"=w387) -> ("error out"=w386:errorcluster)  [unwired: 10 in]
          }
          frame "Busy" {
            n127 = call <vilib>:"Set Busy.vi"("error in (no error)"=w389) -> ("error out"=w388:errorcluster)  [unwired: 9 in, 1 out]
          }
        }
        n128 = call <vilib>:"Add State(s) to Queue__JKI_lib_State_Machine.vi"("State(s) in (\"\")"=w385) -> ("States Out"=w384:string)  [unwired: 14 in]
      }
      frame "UI: Front Panel State" {
        # "Argument"
        n129 = Unbundle By Name(w393) -> ("Core.Current VI Reference"=w392:refnum<vi>)
        n130 = case shown="\"Close\"" w391 {
          tunnel: w395 -> [w401 w414]
          tunnel: [w403 w415] -> w394
          tunnel: w392 -> [w402 w412]
          frame "Open", Default {
            n131 = property class="VI"(reference=w402, error in=w401) -> (reference out=w399:refnum<vi>, error out=w400:errorcluster, "Front Panel.Open"=w398:bool)
            n132 = case shown="False" w398 {
              tunnel: [w406 w409] -> w403
              tunnel: w400 -> [w405 w409]
              tunnel: w399 -> [w404 _]
              frame False {
                n133 = invoke class="VI" method="FP.Open"(reference=w404, error in=w405, "Activate"=TRUE, "State"=T17."Standard") -> (error out=w406:errorcluster)  [unwired: 1 in, 4 out]
              }
              frame True {
              }
            }
          }
          frame "Close" {
            n134 = property class="VI"(reference=w412, error in=w414) -> (reference out=w411:refnum<vi>, error out=w413:errorcluster, "Front Panel.Open"=w410:bool)
            n135 = case shown="True" w410 {
              tunnel: [w416 w419] -> w415
              tunnel: w413 -> [w416 w418]
              tunnel: w411 -> [_ w417]
              frame False {
              }
              frame True {
                n136 = invoke class="VI" method="FP.Close"(reference=w417, error in=w418) -> (error out=w419:errorcluster)  [unwired: 1 in, 2 out]
              }
            }
          }
        }
        n137 = call <vilib>:"Add State(s) to Queue__JKI_lib_State_Machine.vi"("State(s) in (\"\")"=w397) -> ("States Out"=w396:string)  [unwired: 14 in]
      }
      frame "---------- Macro ----------" {
        n138 = call <vilib>:"Add State(s) to Queue__JKI_lib_State_Machine.vi"("State(s) in (\"\")"=w424) -> ("States Out"=w423:string)  [unwired: 14 in]
      }
      frame "Macro: Initialize" {
        n139 = call <vilib>:"Add State(s) to Queue__JKI_lib_State_Machine.vi"("State(s) in Front (\"\")"=w425, "State(s) in (\"\")"=w430) -> ("States Out"=w429:string)  [unwired: 13 in]
      }
      frame "Macro: Exit" {
        # "terminate hs daq loop"
        n140 = Unbundle By Name(w439) -> ("Core.Close Panel on Exit?"=w438:bool)
        n141 = local write "QuitSense"(TRUE ("QuitSense")) -> ()
        n142 = Select(t="UI: Front Panel State >> Close", s=w438, f="") -> (s? t:f=w435:string)
        n143 = call <vilib>:"Add State(s) to Queue__JKI_lib_State_Machine.vi"("State(s) in (\"\")"=w435, "State(s) at Back (\"\")"=w432) -> ("States Out"=w434:string)  [unwired: 13 in]
        n144 = call <vilib>:"Add State(s) to Queue__JKI_lib_State_Machine.vi"("State(s) in Front (\"\")"=w434, "State(s) in (\"\")"=w442) -> ("States Out"=w441:string)  [unwired: 13 in]
      }
      frame "---------- Action ----------" {
        n145 = call <vilib>:"Add State(s) to Queue__JKI_lib_State_Machine.vi"("State(s) in (\"\")"=w447) -> ("States Out"=w446:string)  [unwired: 14 in]
      }
      frame "Action: Wait" {
        n146 = Scan From String(format string="%d", input string=w448, error in=w450, default 1=u32 0) -> (error out=w454:errorcluster, output 1=w453:u32)  [unwired: 1 in, 2 out]
        n147 = call <userlib>:"Wait (ms)__ogtk.vi"("error in (no error)"=w454, "milliseconds to wait"=w453) -> ("error out"=w449:errorcluster)  [unwired: 8 in, 1 out]
        n148 = call <vilib>:"Add State(s) to Queue__JKI_lib_State_Machine.vi"("State(s) in (\"\")"=w458) -> ("States Out"=w457:string)  [unwired: 14 in]
      }
      frame "Action: Terminate AsyncLoop" {
        n149 = Unbundle By Name(w464) -> ("SMQ"=w463:refnum<queue>)
        n150 = Flush Queue(queue=w463) -> (queue out=w462:refnum<queue>)  [unwired: 1 in, 2 out]
        n151 = call <vilib>:"Add State to Queue with vData.vi"("queue in"=w462, "state in"="Macro: Exit", "error in"=w460) -> ("error out"=w459:errorcluster)  [unwired: 9 in, 3 out]
        n152 = call <vilib>:"Add State(s) to Queue__JKI_lib_State_Machine.vi"("State(s) in (\"\")"=w467) -> ("States Out"=w466:string)  [unwired: 14 in]
      }
    }
  }
  n153 = while {
    tunnel: w6 -> [w479]
    shift-right: [w477] -> _
    shift-left: w5 -> [w478]
    shift-right: [w469] -> _
    shift-left: _ -> [w470]
    shift-right: [w471] -> _
    shift-left: DAQLoopSMcase--enum."Init" -> [w475]
    tunnel: w2 -> [w474]
    tunnel: w1 -> [w468]
    stop <- w473 stop-if-true
    n154 = local read "QuitSense"() -> (w472:bool)
    n155 = case shown="\"Run\"" w475 {
      selector: w475 -> [_ w494 w555]
      tunnel: w479 -> [_ w501 w559]
      tunnel: w478 -> [w488 w499 w557]
      tunnel: [w487 w498 w557] -> w477
      tunnel: w474 -> [w489 _ _]
      tunnel: [FALSE _ TRUE] -> w473
      tunnel: w472 -> [w485 w493 _]
      tunnel: [w482 w491 w555] -> w471
      tunnel: w470 -> [_ w496 w556]
      tunnel: [w481 w495 w556] -> w469
      tunnel: w468 -> [_ w490 _]
      frame "Init", Default {
        n156 = register-events(error in=w488, w489) -> (reference out=w481:refnum<event-registration>, error out=w487:errorcluster)  [unwired: 1 in]
        n157 = local write "DAQ Error"(FALSE ("DAQ Error")) -> ()
        n158 = Select(t=DAQLoopSMcase--enum."Stop" ("DaqLoopSMcase"), s=w485, f=DAQLoopSMcase--enum."Run" ("DaqLoopSMcase")) -> (s? t:f=w482:T2)
      }
      frame "Run" {
        n159 = Compound Arithmetic op=AND("HSLoopEn", invert w499) -> (w500:bool)
        n160 = case shown="True" w500 {
          tunnel: w501 -> [_ w542]
          tunnel: w499 -> [w504 w536]
          tunnel: [w503 w537] -> w498
          tunnel: w496 -> [w502 w538]
          tunnel: [w502 w538] -> w495
          tunnel: w490 -> [_ w525]
          frame False {
            n161 = event shown="[1] <PrivateAsync Ev>: User Event" {
              selector: w502 -> [_ _]
              dyn-events: _ -> [_ _]
              timeout: 500 ("milliseconds to wait") -> [_ _]
              tunnel: w504 -> [w506 w508]
              tunnel: [w506 w507] -> w503
              event Timeout {
                n162 = event-data() -> ()  [unwired: 1 in, 1 out]
              }
              event User Event {
                n163 = event-data() -> ("vData"=w509:variant, "CmdMsg"=w511:string)  [unwired: 1 in, 1 out]
                n164 = Scan From String(format string="%s", input string=w511, default 1=PrivateAsynEv_DAQ_Engine--enum."PrivDAQ.ClearDAQError" ("PrivAsyncCmd")) -> (output 1=w513:T15)  [unwired: 2 in, 3 out]
                n165 = case shown="\"PrivDAQ.ClearDAQError\"" w513 {
                  tunnel: w509 -> [_ _]
                  tunnel: w508 -> [w514 _]
                  tunnel: [w514 w516] -> w507
                  frame Default {
                  }
                  frame "PrivDAQ.ClearDAQError" {
                    w516 = errorcluster {"status"=FALSE, "code"=0, "source"=""} ("error constant")
                    n166 = call "FG - DAQ Error Cluster.vi"("action (Get)"=TD_GetSet_ActionSelect--enum."Set", "error"=w516) -> ()  [unwired: 9 in, 1 out]
                  }
                }
              }
            }
          }
          frame True {
            # "provide an offset if in demo mode"
            n167 = global read "GBL System.vi" "RIO Device"() -> (w517:T22)
            n168 = call "Compute Expected DAQ Loop Interval.vi"("Measurement config"="MeasSet", "error in (no error)"=w536, "MinDemoWait (20ms)"=u32 20, "MaxDemoWait (10000)"=u32 10000, "DemoMode"=w525) -> ("error out"=w519:errorcluster, "WaitFunction Value"=→"WaitFunction Value":u32, "Computed Loop Interval"=→"computed loop time":u32)  [unwired: 4 in]
            n169 = disable-structure shown="Enabled" {
              disable-tunnel: "MeasSet" -> [w547 w551]
              disable-tunnel: [w546 w550] -> w523
              disable-tunnel: [w545 w548] -> w522
              disable-tunnel: [w544 w549] -> w521
              disable-tunnel: w517 -> [w543 _]
              frame Disabled {
                n170 = call "cRIO HOST.vi"("resource name"=w543, "MeasSet"=w547) -> ("Start time"=w545:timestamp, "data 9775x2"=w544:dbl[], "data 9215"=w546:dbl[])  [unwired: 4 in, 3 out]
              }
              frame Enabled {
                n171 = call "cRIO HOST_Simulation.vi"("MeasSet"=w551) -> ("current time"=w548:timestamp, "9775"=w549:dbl[], "9215"=w550:dbl[])  [unwired: 8 in]
              }
            }
            n172 = Add(x=1.0, y=w523) -> (x+y=w531:dbl[])
            n173 = Add(x=2.0, y=w521) -> (x+y=w529:dbl[])
            n174 = Select(t=w531, s=w525, f=w523) -> (s? t:f=w526:dbl[])
            n175 = Select(t=w529, s=w525, f=w521) -> (s? t:f=w527:dbl[])
            n176 = call <userlib>:"Wait (ms)__ogtk.vi"("error in (no error)"=w519, "milliseconds to wait"=u32 100) -> ("error out"=w518:errorcluster)  [unwired: 8 in, 1 out]
            n177 = Bundle By Name(cluster=T20 {"Module1-2_9775"={"TS"=timestamp(0 s since 1904-01-01), "ScanArray"=[]}, "Module 3-4_9215"={"TS"=timestamp(0 s since 1904-01-01), "ScanArray"=[]}} ("RawDAQData"), "Module 3-4_9215.ScanArray"=w526, "Module 3-4_9215.TS"=w522, "Module1-2_9775.ScanArray"=w527, "Module1-2_9775.TS"=w522) -> (w540:T20)
            n178 = Enqueue Element(queue=w542, element=w540) -> (timed out?=→"DaqQ Timeout":bool, error out=w537:errorcluster)  [unwired: 2 in, 1 out]
            n179 = case shown="No Error" w518 {
              tunnel: w537 -> [w552 _]
              frame No Error {
                n180 = case shown="No Error" w552 {
                  selector: w552 -> [_ w553]
                  frame No Error {
                  }
                  frame Error {
                    n181 = call "FG - DAQ Error Cluster.vi"("action (Get)"=TD_GetSet_ActionSelect--enum."Set", "error"=w553) -> ()  [unwired: 9 in, 1 out]
                  }
                }
              }
              frame Error {
              }
            }
          }
        }
        n182 = Select(t=DAQLoopSMcase--enum."Stop", s=w493, f=w494) -> (s? t:f=w491:T2)
      }
      frame "Stop" {
        n183 = Flush Queue(queue=w559) -> ()  [unwired: 1 in, 3 out]
        n184 = Unregister For Events(event registration refnum=w556) -> ()  [unwired: 1 in, 1 out]
      }
    }
    n185 = Unbundle By Name(w477) -> ("status"=→"DAQ Error":bool)
  }
  n186 = Merge Errors(w9, w8) -> ()  [unwired: 1 out]
